vi "J-KEM_subVI_no_control 2017-11-10.vi"(10 "Address in":T1) -> (0 "Temp (C)":dbl format="%#_6f", 3 "Address out":T1)   [LabVIEW 2014]
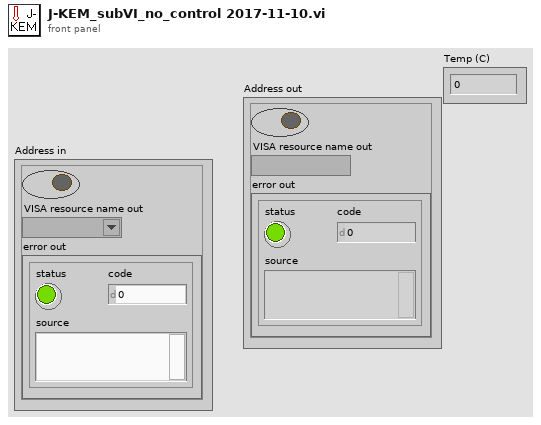
[diagram p1: front panel]
types:
  T1 = cluster{"Boolean":bool, "VISA resource name out":refnum<visa-resource-name>, "error out":errorcluster}
  T2 = cluster{bool, "VISA resource name out":refnum<visa-resource-name>, "error out":errorcluster}
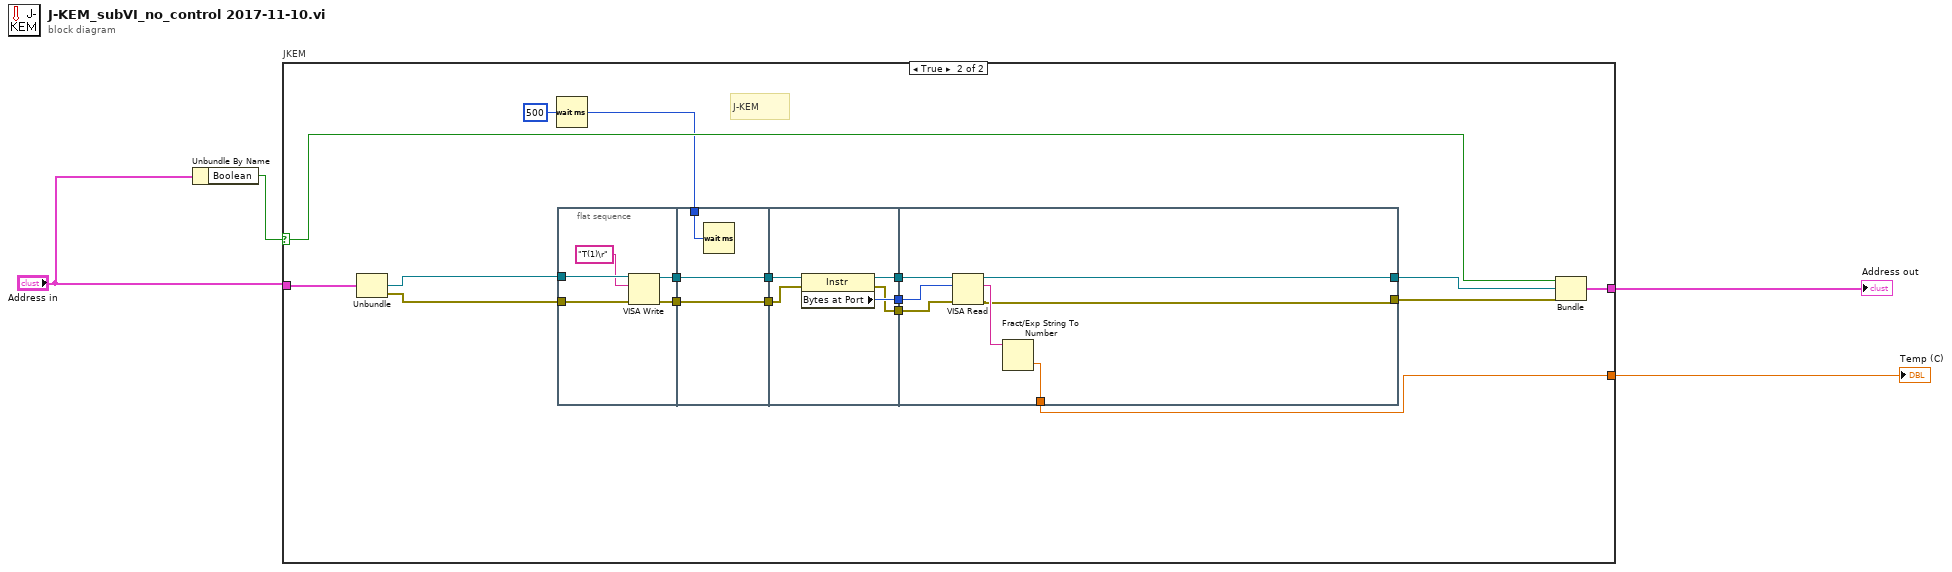
[diagram p0: block diagram]
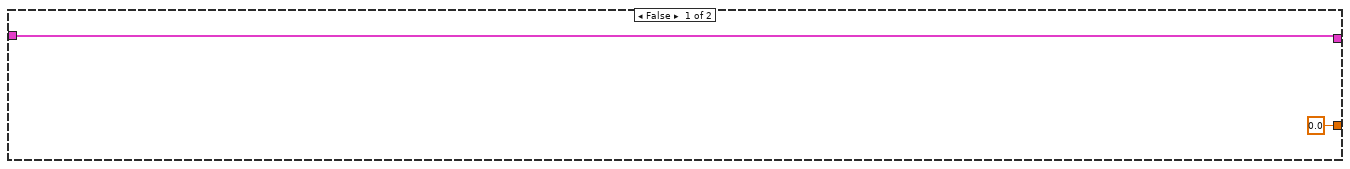
[diagram p2: hidden frame]
diagram:
  n1 = Unbundle By Name("Address in") -> ("Boolean"=w1:bool)
  n2 = case "JKEM" shown="True" w1 {
    selector: w1 -> [_ w17]
    tunnel: "Address in" -> [w6 w20]
    tunnel: [w6 w18] -> w4
    tunnel: [0.0 w7] -> w3
    frame False {
    }
    frame True {
      w8 = u32 500 ("milliseconds to wait")
      # "J-KEM"
      n3 = Unbundle(w20) -> ("VISA resource name out"=w19:refnum<visa-resource-name>, "error out"=w16:errorcluster)  [unwired: 1 out]
      n4 = Wait (ms)(milliseconds to wait=w8) -> ()  [unwired: 1 out]
      n5 = flat-sequence {
        tunnel: w19 -> [w27]
        tunnel: w16 -> [w26]
        tunnel: [w24] -> w15
        tunnel: [w23] -> w14
        tunnel: w8 -> [w30]
        tunnel: [w29] -> w13
        tunnel: w15 -> [w29]
        tunnel: w14 -> [w28]
        tunnel: [w28] -> w12
        tunnel: w13 -> [w35]
        tunnel: w12 -> [w34]
        tunnel: [w33] -> w11
        tunnel: [w32] -> w10
        tunnel: [w31] -> w9
        tunnel: [w42] -> w21
        tunnel: [w36] -> w22
        tunnel: [w37] -> w7
        tunnel: w9 -> [w39]
        tunnel: w10 -> [w40]
        tunnel: w11 -> [w41]
        frame #0 {
          n6 = VISA Write(VISA resource name=w27, write buffer="T(1)\r", error in (no error)=w26) -> (VISA resource name out=w24:refnum<visa-resource-name>, error out=w23:errorcluster)  [unwired: 1 out]
        }
        frame #1 {
          n7 = Wait (ms)(milliseconds to wait=w30) -> ()  [unwired: 1 out]
        }
        frame #2 {
          n8 = property class="Instr"(reference=w35, error in=w34) -> (reference out=w33:refnum<visa-resource-name>, error out=w31:errorcluster, "Bytes at Port"=w32:u32)
        }
        frame #3 {
          n9 = VISA Read(VISA resource name=w41, byte count=w40, error in (no error)=w39) -> (VISA resource name out=w42:refnum<visa-resource-name>, read buffer=w38:string, error out=w36:errorcluster)  [unwired: 1 out]
          n10 = Fract/Exp String To Number(string=w38) -> (number=w37:dbl)  [unwired: 3 in, 1 out]
        }
      }
      n11 = Bundle(w17, "VISA resource name out"=w21, "error out"=w22) -> (w18:T2)  [unwired: 1 in]
    }
  }
  "Address out" <- w4
  "Temp (C)" <- w3
